vi "Attemp Arduino connection.vi"(8 "error in (no error)":errorcluster, 11 "COM port in":refnum<visa-resource-name>) -> (0 "error out":errorcluster, 3 "COM port out":refnum<visa-resource-name>)   [LabVIEW 2020]
doc: "Attempts a connection to an Arduino with LED Controller script loaded. Returns error 5004 if the device at the specified port is not the intended driver."
uses:
  eccd119d-ebd3-48f1-821d-f99a79d32177.vi
  <vilib>/Utility/error.llb/Error Cluster From Error Code.vi
  <vilib>/Instr/_visa.llb/VISA Configure Serial Port (Instr).vi
  <vilib>/ErrorRing/Error Ring.xnode
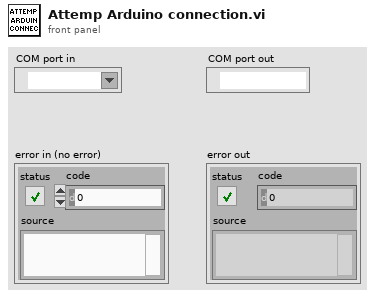
[diagram p1: front panel]
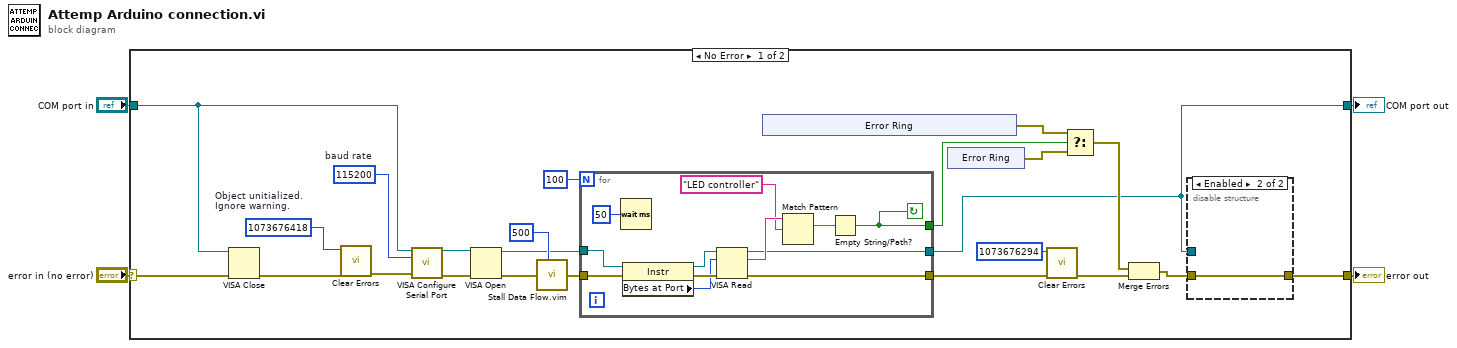
[diagram p0: block diagram]
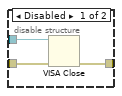
[diagram p2: hidden frame]
diagram:
  n1 = case shown="No Error" "error in (no error)" {
    selector: "error in (no error)" -> [w27 w51]
    tunnel: "COM port in" -> [w18 w50]
    tunnel: [w21 w51] -> w3
    tunnel: [w9 w50] -> w1
    frame No Error {
      w7 = 1073676418  # Object unitialized. Ignore warning.
      w26 = u32 115200  # baud rate
      n2 = VISA Close(VISA resource name=w18, error in (no error)=w27) -> (error out=w6:errorcluster)
      n3 = call <vilib>:"Clear Errors.vi"("error in (no error)"=w6, "specific error code to clear (0: all)"=w7) -> ("error out"=w5:errorcluster)  [unwired: 4 in, 1 out]
      n4 = call-poly "VISA Configure Serial Port"("VISA resource name"=w18, "baud rate (9600)"=w26, "error in (no error)"=w5) -> ("VISA resource name out"=w12:refnum<visa-resource-name>, "error out"=w20:errorcluster)  [unwired: 11 in]
      n5 = VISA Open(error in (no error)=w20, VISA resource name=w12) -> (VISA resource name=w11:refnum<visa-resource-name>, error out=w13:errorcluster)  [unwired: 3 in]
      n6 = call "Stall Data Flow.vim"("value in"=w13, "milliseconds to wait"=u32 500) -> ("value out"=w17:errorcluster)  [unwired: 1 out]
      n7 = for {
        N: 100 -> [_]
        tunnel: w11 -> [w37]
        tunnel: [w30] -> w14
        tunnel: w17 -> [w34]
        tunnel: [w39] -> w19
        tunnel: [w28] -> w9
        stop <- w30 continue-if-true
        n8 = Wait (ms)(milliseconds to wait=u32 50) -> ()  [unwired: 1 out]
        n9 = property class="Instr"(reference=w37, error in=w34) -> (reference out=w36:refnum<visa-resource-name>, error out=w38:errorcluster, "Bytes at Port"=w35:u32)
        n10 = VISA Read(VISA resource name=w36, byte count=w35, error in (no error)=w38) -> (VISA resource name out=w28:refnum<visa-resource-name>, read buffer=w32:string, error out=w39:errorcluster)  [unwired: 1 out]
        n11 = Match Pattern(string=w32, regular expression="LED controller") -> (match substring=w29:string)  [unwired: 1 in, 3 out]
        n12 = Empty String/Path?(string/path=w29) -> (empty?=w30:bool)
      }
      n13 = xnode "Error Ring"() -> ("error out"=w24:errorcluster)
      n14 = xnode "Error Ring"() -> ("error out"=w25:errorcluster)
      n15 = call <vilib>:"Clear Errors.vi"("error in (no error)"=w19, "specific error code to clear (0: all)"=1073676294) -> ("error out"=w10:errorcluster)  [unwired: 4 in, 1 out]
      n16 = Select(t=w24, s=w14, f=w25) -> (s? t:f=w23:errorcluster)
      n17 = Merge Errors(w23, w10) -> (w22:errorcluster)
      n18 = disable-structure shown="Enabled" {
        disable-tunnel: w22 -> [w48 w49]
        disable-tunnel: [w47 w49] -> w21
        disable-tunnel: w9 -> [w46 _]
        frame Disabled {
          n19 = VISA Close(VISA resource name=w46, error in (no error)=w48) -> (error out=w47:errorcluster)
        }
        frame Enabled {
        }
      }
    }
    frame Error {
    }
  }
  "error out" <- w3
  "COM port out" <- w1
